vi "CRC Test.vi"() -> ()   [LabVIEW 2014]
uses:
  MAVLink CRC v2 Generate.vi
  MAVLink CRC v2 Check.vi
panel:
  out "Message w/ CRC":u8[](array[numeric]) format="%x"
  out "output packet":u8[](array[numeric]) format="%x"
  out "CRC Gen MSG Match":bool
  out "CRC good":bool
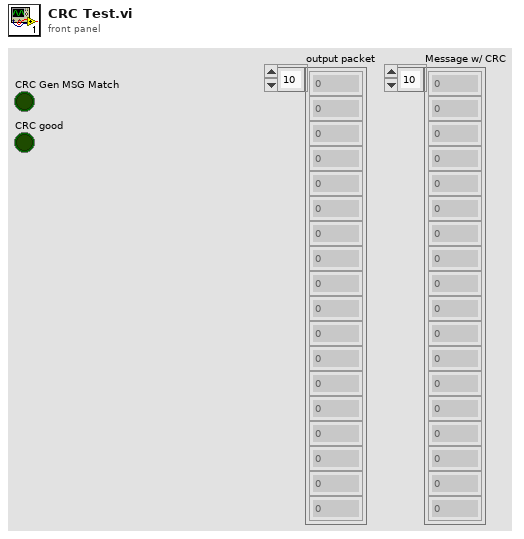
[diagram p1: front panel]
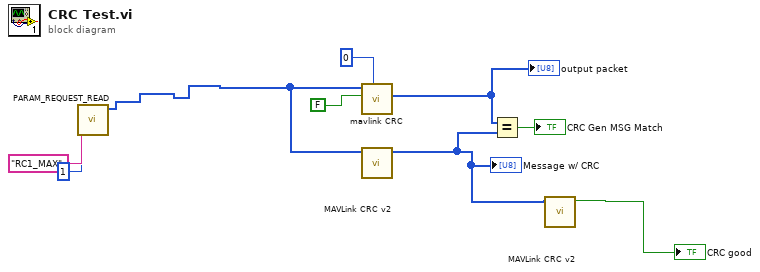
[diagram p0: block diagram]
diagram:
  n1 = call "PARAM_REQUEST_READ.vi"("Target System and Target Component"=u8 1, "param_id"="RC1_MAX") -> ("MAVLink Message"=w3:u8[])  [unwired: 9 in]
  n2 = call "mavlink CRC.vi"("AircraftID"=u8 0, "Check (T)/ Generate (F)"=FALSE, "byte array input"=w3) -> ("output packet"=w7:u8[])  [unwired: 7 in, 1 out]
  "output packet" <- w7
  n3 = call-poly "MAVLink CRC v2.vi"("Message"=w3) -> ("Message w/ CRC"=w5:u8[])  [unwired: 10 in]
  "Message w/ CRC" <- w5
  n4 = Equal?(x=w7, y=w5) -> (x = y?=→"CRC Gen MSG Match":bool)
  n5 = call-poly "MAVLink CRC v2.vi"("Message"=w5) -> ("CRC good"=→"CRC good":bool)  [unwired: 10 in]
